vi "Extract Image.vi"() -> ()   [LabVIEW 2014]
doc: "This example shows how to extract one region of an image into a new image."
uses:
  <vilib>/vision/NI_Vision_Development_Module.lvlib
panel:
  in  "Optional Rectangle":i32[](array[numeric])=[192, 108, 374, 256]
  out "Extracted Image":T1(plugin-control)
  out "Image Source":T1(plugin-control)
  in  "Y Step":i32=3 min=1
  in  "X Step":i32=2 min=1
  # "Overview: Demonstrates how to extract a portion of an image using the IMAQ Extract VI.\nRequirements: NI Vision Development Module\nInstructions: Run the VI."
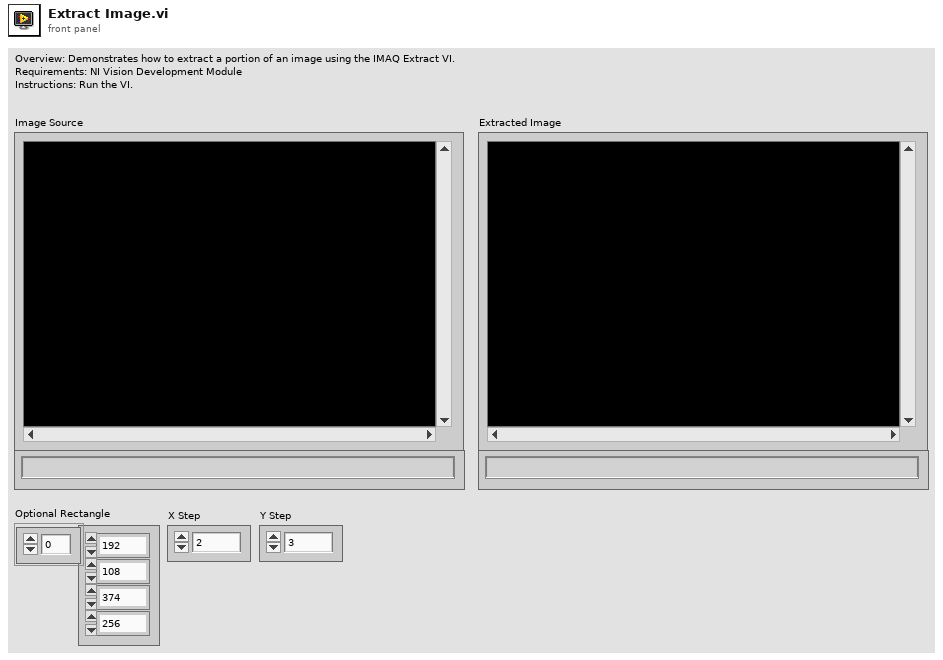
[diagram p1: front panel]
types:
  T1 = typedef "IMAQ Image.ctl" = refnum<image>
  T2 = typedef "Image Type" = u32
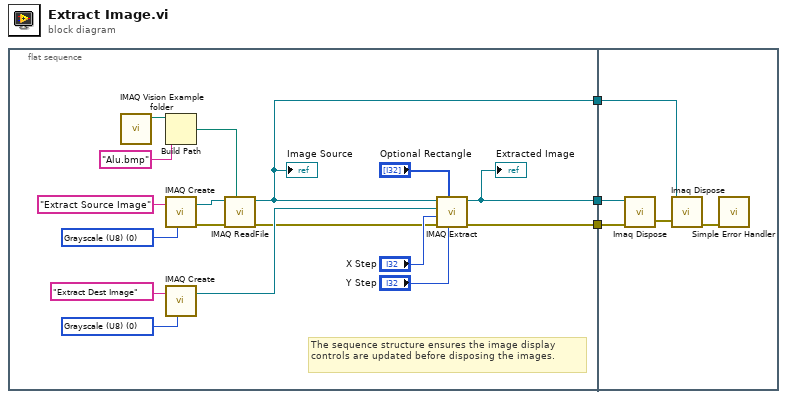
[diagram p0: block diagram]
diagram:
  n1 = flat-sequence {
    tunnel: [w12] -> w3
    tunnel: [w11] -> w2
    tunnel: [w5] -> w1
    tunnel: w3 -> [w22]
    tunnel: w2 -> [w23]
    tunnel: w1 -> [w21]
    frame #0 {
      w7 = T2 0 items=["Grayscale (U8)", "Grayscale (I16)", "Grayscale (SGL)", "Complex (CSG)", "RGB (U32)", "HSL (U32)", "RGB (U64)", "Grayscale (U16)"] ("Image Type")
      w8 = T2 0 items=["Grayscale (U8)", "Grayscale (I16)", "Grayscale (SGL)", "Complex (CSG)", "RGB (U32)", "HSL (U32)", "RGB (U64)", "Grayscale (U16)"] ("Image Type")
      # "The sequence structure ensures the image display controls are updated before disposing the images."
      n2 = call "IMAQ Vision Example folder.vi"() -> ("Example Image Path"=w19:path)  [unwired: 11 in]
      n3 = Build Path(base path=w19, name or relative path="Alu.bmp") -> (appended path=w14:path)
      n4 = call "IMAQ Create"("Image Name"="Extract Source Image", "Image Type"=w8) -> ("New Image"=w16:T1, "error out"=w15:errorcluster)  [unwired: 3 in]
      n5 = call "IMAQ Create"("Image Name"="Extract Dest Image", "Image Type"=w7) -> ("New Image"=w13:T1)  [unwired: 3 in, 1 out]
      n6 = call "IMAQ ReadFile"("File Path"=w14, "error in (no error)"=w15, "Image"=w16) -> ("error out"=w9:errorcluster, "Image Out"=w5:T1)  [unwired: 4 in, 3 out]
      "Image Source" <- w5
      n7 = call "IMAQ Extract"("Y Step Size"="Y Step", "Optional Rectangle"="Optional Rectangle", "error in (no error)"=w9, "X Step Size"="X Step", "Image Dst"=w13, "Image Src"=w5) -> ("error out"=w12:errorcluster, "Image Dst Out"=w11:T1)  [unwired: 4 in]
      "Extracted Image" <- w11
    }
    frame #1 {
      n8 = call "Imaq Dispose"("Image"=w23, "error in (no error)"=w22) -> ("error out"=w24:errorcluster)  [unwired: 4 in]
      n9 = call "Imaq Dispose"("Image"=w21, "error in (no error)"=w24) -> ("error out"=w25:errorcluster)  [unwired: 4 in]
      n10 = call <vilib>:"Simple Error Handler.vi"("error in (no error)"=w25) -> ()  [unwired: 4 in, 5 out]
    }
  }
